vi "constructor.vi"   [LabVIEW 2014]
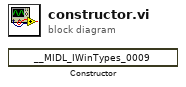
[diagram p0: block diagram]
diagram:
  n1 = constructor class="__MIDL_IWinTypes_0009"() -> ()  [unwired: 3 in, 3 out]
